vi "SwissSPAD Live_Init Internal Data Storage.vi"(8 "Error In":errorcluster) -> (0 "Error Out":errorcluster)   [LabVIEW 2021]
uses:
  SwissSPAD Live_Internal Data List.ctl
panel:
  in  "SwissSPAD Live Internal Data List":T1
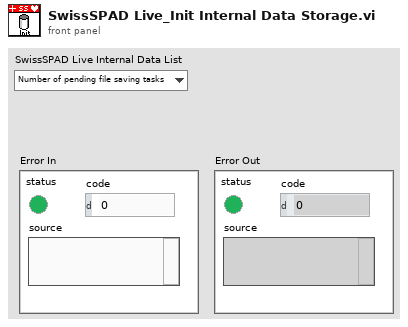
[diagram p1: front panel]
types:
  T1 = typedef "SwissSPAD Live_Internal Data List.ctl" = enum16{"Number of pending file saving tasks", "File Saving Tasks Information", "Current Image ROI Information", "# FPGA Reset Attempts", "Histogram Cursor Locations", "Histogram Window is Open"}
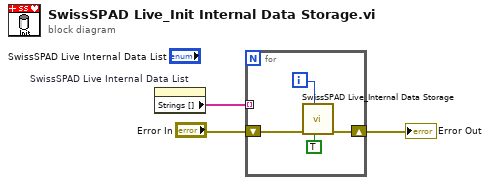
[diagram p0: block diagram]
diagram:
  n1 = property on="SwissSPAD Live Internal Data List" class="Enum (strict)"() -> ("Strings []"=w3:string[])  [unwired: 2 in, 2 out]
  n2 = for {
    tunnel: w3 -> [_] mode=indexing
    shift-right: [w4] -> w1
    shift-left: "Error In" -> [w5]
    i -> [w7]
    n3 = call "SwissSPAD Live_Internal Data Storage.vi"("Get(F)/Set"=TRUE, "SS2 Live Data"=w7, "Error In"=w5) -> ("Error Out"=w4:errorcluster)  [unwired: 6 in, 2 out]
  }
  "Error Out" <- w1
